vi "trim_whitespaces.vi"() -> ()   [LabVIEW 2019]
panel:
  out "length 2":i32
  out "length":i32
  out "trimmed string":string
  out "concatenated string":string
  in  "string 2":string="WORLD             "
  in  "string":string="     hello"
  # "1. This program will print hello in upper case (HELLO)and world in lower case(world) \n2. Then it will concatenate the two strings and will print the string with the length\n3. It will remove the whitespaces and will print the strings with length"
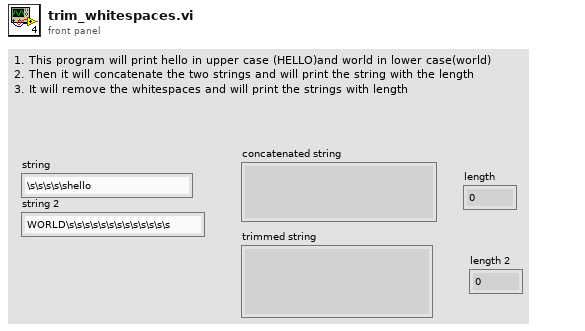
[diagram p1: front panel]
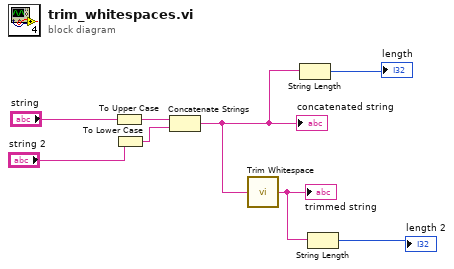
[diagram p0: block diagram]
diagram:
  n1 = To Upper Case(1:"string") -> (0:w8:string)
  n2 = To Lower Case(string="string 2") -> (all lower case string=w7:string)
  n3 = Concatenate Strings(w8, w7) -> (w4:string)
  "concatenated string" <- w4
  n4 = call <vilib>:"Trim Whitespace.vi"("string"=w4) -> ("trimmed string"=w3:string)  [unwired: 1 in]
  "trimmed string" <- w3
  n5 = String Length(string=w4) -> (length=→"length":i32)
  n6 = String Length(string=w3) -> (length=→"length 2":i32)
